vi "BRig_dataRT_stats__FreeReward_c_L.vi"() -> (2 "output_FreeReward_c_L":i32)   [LabVIEW 2014]
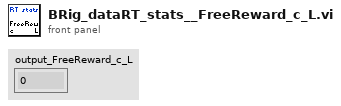
[diagram p1: front panel]
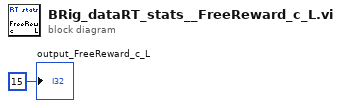
[diagram p0: block diagram]
diagram:
  "output_FreeReward_c_L" <- 15 ("output_iBlock")
